vi "Scaled Window for N Chan.vi"(8 "error in (no error)":errorcluster, 9 "window parameter":dbl=nan, 10 "window":T1 items=["Rectangle"=0, "Hanning"=1, "Hamming"=2, "Blackman-Harris"=3, "Exact Blackman"=4, "Blackman"=5, "Flat Top"=6, "4 Term B-Harris "=7, "7 Term B-Harris"=8, "Low Sidelobe"=9, "Blackman Nuttall"=11, "Triangle"=30, "Bartlett-Hanning"=31, "Bohman"=32, "Parzen"=33, "Welch"=34, "Kaiser"=60, "Dolph-Chebyshev"=61, "Gaussian"=62], 11 "signals in":waveform(dbl)[](array[waveform])) -> (0 "error out":errorcluster, 2 "window constants":cluster{"eq noise BW":dbl, "coherent gain":dbl} {"coherent gain" format="%.6f"; "eq noise BW" format="%.6f"}, 3 "signals out":waveform(dbl)[](array[waveform]))   [LabVIEW 2020, in "NI_MAPro.lvlib"]
doc: "Applies a scaled window to the time-domain signal and outputs window constants for further analysis. Wire data to the <B>signal in</B> input to determine the polymorphic instance to use or manually select the instance."
uses:
  NI_MAPro.lvlib
  windowTd.ctl
  NI_MABase.lvlib
  NI_AALPro.lvlib
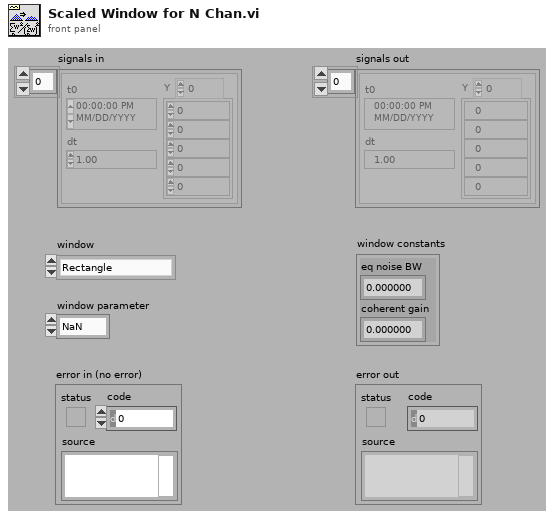
[diagram p1: front panel]
types:
  T1 = typedef "NI_AALPro.lvlib/windowTd.ctl" = u32
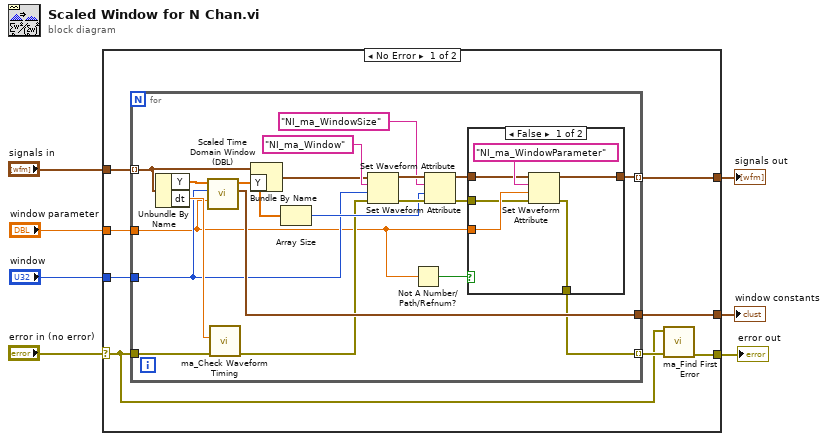
[diagram p0: block diagram]
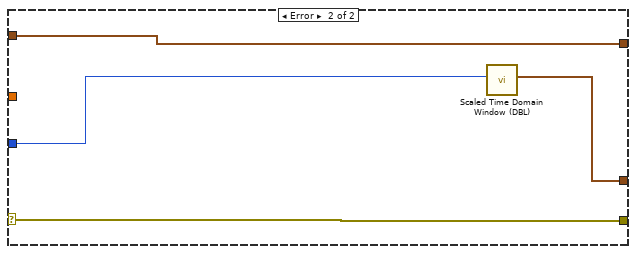
[diagram p3: hidden frame]
diagram:
  n1 = case shown="No Error" "error in (no error)" {
    selector: "error in (no error)" -> [w9 w44]
    tunnel: "window" -> [w15 w45]
    tunnel: [w14 w46] -> w6
    tunnel: [w12 w47] -> w4
    tunnel: "signals in" -> [w13 w47]
    tunnel: [w10 w44] -> w2
    tunnel: "window parameter" -> [w8 _]
    frame No Error {
      n2 = for {
        tunnel: w15 -> [w20]
        tunnel: [w35] -> w14
        tunnel: w13 -> [w32] mode=indexing
        tunnel: [w22] -> w12 mode=indexing
        tunnel: w9 -> [w33]
        tunnel: [w19] -> w11 mode=indexing
        tunnel: w8 -> [w17]
        n3 = Unbundle By Name(w32) -> ("Y"=w34:dbl[], "dt"=w31:dbl)
        n4 = call "Scaled Time Domain Window (DBL).vi"("window parameter"=w17, "window"=w20, "X"=w34) -> ("window properties"=w35:cluster{"eq noise BW":dbl, "coherent gain":dbl}, "Windowed X"=w21:dbl[])  [unwired: 6 in, 1 out]
        n5 = call "ma_Check Waveform Timing.vi"("error in (no error)"=w33, "dt"=w31) -> ("error out"=w18:errorcluster)  [unwired: 8 in, 1 out]
        n6 = Bundle By Name(cluster=w32, "Y"=w21) -> (w23:waveform(dbl))
        n7 = Array Size(array=w21) -> (size(s)=w26:i32)
        n8 = Set Waveform Attribute(4:w18, 5:w20, 6:"NI_ma_Window" ("name"), 7:w23) -> (0:w27:errorcluster, 3:w30:waveform(dbl))  [unwired: 1 out]
        n9 = Not A Number/Path/Refnum?(number/path/refnum=w17) -> (NaN/Path/Refnum?=w16:bool)
        n10 = Set Waveform Attribute(4:w27, 5:w26, 6:"NI_ma_WindowSize" ("name"), 7:w30) -> (0:w24:errorcluster, 3:w25:waveform(dbl))  [unwired: 1 out]
        n11 = case shown="False" w16 {
          tunnel: w25 -> [w40 w43]
          tunnel: [w39 w43] -> w22
          tunnel: w17 -> [w38 _]
          tunnel: [w37 w42] -> w19
          tunnel: w24 -> [w36 w42]
          frame False {
            n12 = Set Waveform Attribute(4:w36, 5:w38, 6:"NI_ma_WindowParameter" ("name"), 7:w40) -> (0:w37:errorcluster, 3:w39:waveform(dbl))  [unwired: 1 out]
          }
          frame True {
          }
        }
      }
      n13 = call "ma_Find First Error.vi"("error array in"=w11, "error in 1 (no error)"=w9) -> ("error out"=w10:errorcluster)  [unwired: 5 in]
    }
    frame Error {
      n14 = call "Scaled Time Domain Window (DBL).vi"("window"=w45) -> ("window properties"=w46:cluster{"eq noise BW":dbl, "coherent gain":dbl})  [unwired: 8 in, 2 out]
    }
  }
  "window constants" <- w6
  "error out" <- w2
  "signals out" <- w4
